vi "Delay.vi"(8 "error in (no error)":errorcluster, 11 "pre-read delay(ms)":i16) -> (0 "error out":errorcluster)   [LabVIEW 2022 SP3, in "Serial-Com-Libraries.lvlib" / "Serial Base.lvclass"]
doc: "wait the amount of miliseconds specified in the input\nNote: if delay == -1 then it will not delay\n-------------------------------------------\n<b>pre-read delay(ms)</b>: miliseconds to wait, type <b>-1</b> to not wait"
uses:
  Serial Base.lvclass
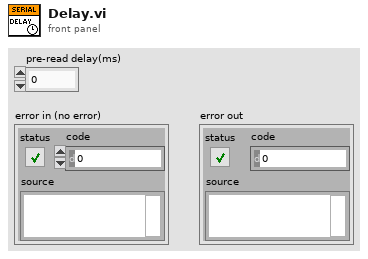
[diagram p1: front panel]
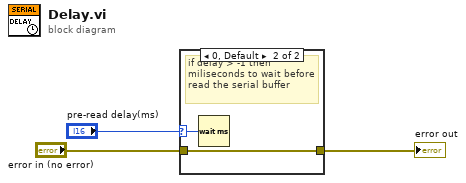
[diagram p0: block diagram]
diagram:
  n1 = case shown="0, Default" "pre-read delay(ms)" {
    selector: "pre-read delay(ms)" -> [_ w5]
    tunnel: "error in (no error)" -> [w4 w6]
    tunnel: [w4 w6] -> w1
    frame -1 {
      # "-1 = not delay"
    }
    frame 0, Default {
      # "if delay > -1 then miliseconds to wait before read the serial buffer"
      n2 = Wait (ms)(milliseconds to wait=w5) -> ()  [unwired: 1 out]
    }
  }
  "error out" <- w1
